vi "Connect Route.vi"(4 "Promise in":refnum<class "Promise.lvclass">, 6 "Mux Index":i32, 8 "error in (no error)":errorcluster, 9 "Output":i32, 10 "Input":i32, 11 "MuxActor in":refnum<class "MuxActor.lvclass">) -> (0 "error out":errorcluster, 3 "MuxActor out":refnum<class "MuxActor.lvclass">)   [LabVIEW 2022 SP3, in "VideoMux.lvlib" / "MuxActor.lvclass"]
uses:
  MuxActor.lvclass
  <vilib>/IlluminatedG/IG Promises/Promises/Promise/Promise.lvclass
  MuxActor.lvclass/MuxActor.ctl
  MuxRoute Value/MuxRoute Value.lvclass
  C:/Program Files (x86)/National Instruments/LabVIEW 2022/vi.lib/IlluminatedG/IG Promises/Promises/Value/Value.lvclass
  Mux/Mux.lvclass
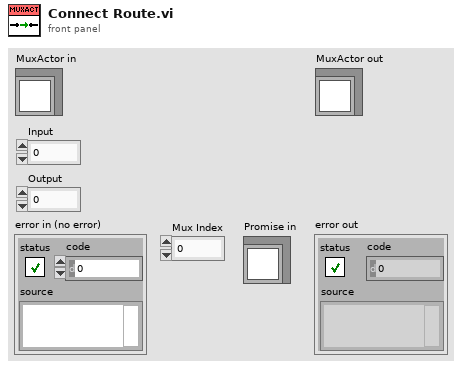
[diagram p1: front panel]
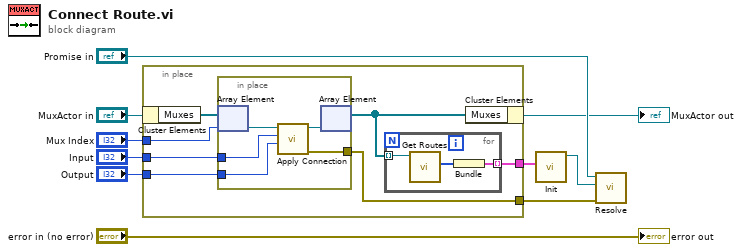
[diagram p0: block diagram]
diagram:
  n1 = in-place {
    in-place-border: "Mux Index" -> [w16]
    in-place-border: "Input" -> [w15]
    in-place-border: "Output" -> [w14]
    in-place-border: [w12] -> w4
    in-place-border: [w11] -> w5
    n2 = in-place-cluster #1("MuxActor in") -> ("Muxes"=w17:refnum<class "Mux.lvclass">[])
    n3 = in-place {
      in-place-border: w15 -> [w24]
      in-place-border: w14 -> [w23]
      in-place-border: [w21] -> w12
      n4 = in-place-array #2(w17, w16) -> (w25:refnum<class "Mux.lvclass">)
      n5 = call-dynamic "Apply Connection.vi"("Output Index"=w23, "Input Index"=w24, "Mux in"=w25) -> ("error out"=w21:errorcluster, "Mux out"=w22:refnum<class "Mux.lvclass">)  [unwired: 7 in]
      n6 = in-place-array #2(w22) -> (w13:refnum<class "Mux.lvclass">[])  [unwired: 1 out]
    }
    n7 = for {
      tunnel: w13 -> [w20] mode=indexing
      tunnel: [w18] -> w11 mode=indexing
      n8 = call "Get Routes.vi"("Mux in"=w20) -> ("Routes"=w19:i32[])  [unwired: 8 in, 2 out]
      n9 = Bundle("Routes"=w19) -> (w18:cluster{"Routes":i32[]})  [unwired: 1 in]
    }
    n10 = in-place-cluster #1("Muxes"=w13) -> (→"MuxActor out":refnum<class "MuxActor.lvclass">)
  }
  n11 = call "Init.vi"("Muxes"=w5) -> ("MuxRoute Value out"=w3:refnum<class "MuxRoute Value.lvclass">)  [unwired: 9 in, 1 out]
  n12 = call <vilib>:"Resolve.vi"("error in (no error)"=w4, "Result"=w3, "Promise in"="Promise in") -> ()  [unwired: 7 in, 2 out]
  "error out" <- "error in (no error)"
